vi "NicmosInitSerial.vi"(0 "error in (no error)":errorcluster caption="entrée d'erreur", 5 "Port Nicmos":refnum<visa-resource-name>="COM1") -> (3 "error out":errorcluster caption="sortie d'erreur")   [LabVIEW 2009]
uses:
  NicmosGlobal.vi
  <vilib>/Instr/_visa.llb/VISA Configure Serial Port (Serial Instr).vi
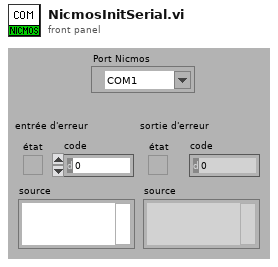
[diagram p1: front panel]
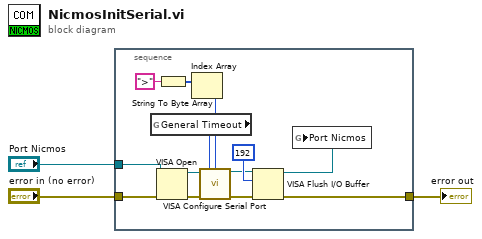
[diagram p0: block diagram]
diagram:
  n1 = stacked-sequence {
    tunnel: [w4] -> w1
    tunnel: "Port Nicmos" -> [w6]
    tunnel: "error in (no error)" -> [w8]
    frame #0 {
      n2 = global read "NicmosGlobal.vi" "General Timeout"() -> (w12:u32)
      n3 = VISA Open(error in (no error)=w8, VISA resource name=w6) -> (VISA resource name=w5:refnum<visa-resource-name>, error out=w7:errorcluster)  [unwired: 3 in]
      n4 = String To Byte Array(string=">") -> (unsigned byte array=w15:u8[])
      n5 = Index Array(array=w15) -> (element=w13:u8)  [unwired: 1 in]
      n6 = call-poly "VISA Configure Serial Port"("VISA resource name"=w5, "timeout (10sec)"=w12, "termination char\n(0xA = '\\n' = LF)"=w13, "error in (no error)"=w7) -> ("VISA resource name out"=w11:refnum<visa-resource-name>, "error out"=w10:errorcluster)  [unwired: 10 in]
      n7 = VISA Flush I/O Buffer(VISA resource name=w11, mask (16)=u16 192, error in (no error)=w10) -> (VISA resource name out=w9:refnum<visa-resource-name>, error out=w4:errorcluster)
      n8 = global write "NicmosGlobal.vi" "Port Nicmos"(w9) -> ()
    }
  }
  "error out" <- w1
